vi "mapown org loop.vi"() -> ()   [LabVIEW 2011]
panel:
  in  "Close":bool
  in  "Update View":bool
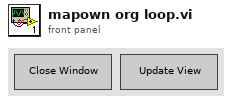
[diagram p1: front panel]
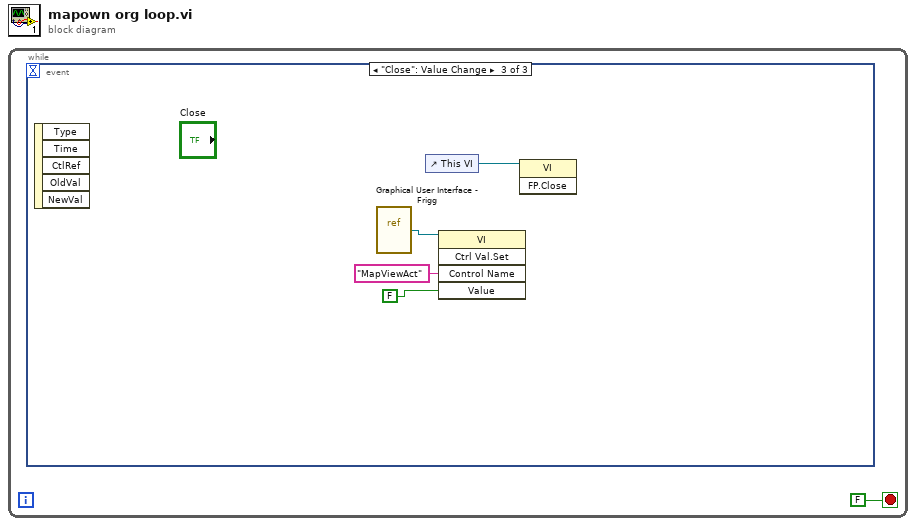
[diagram p0: block diagram]
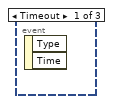
[diagram p2: hidden frame]
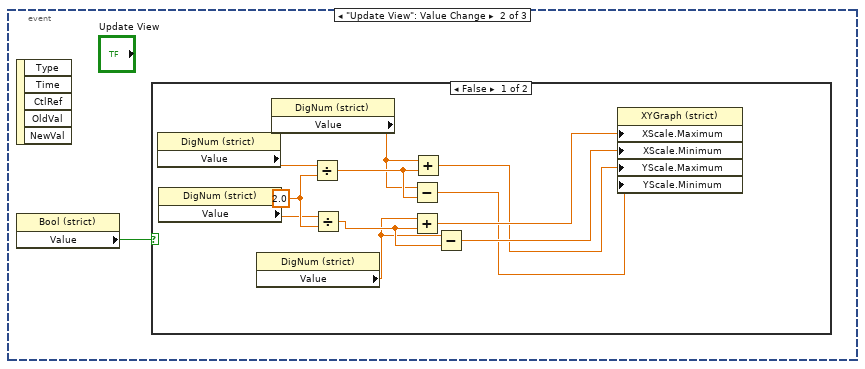
[diagram p3: hidden frame]
diagram:
  n1 = while {
    stop <- FALSE stop-if-true
    n2 = event shown="[2] \"Close\": Value Change" {
      selector: _ -> [_ _ _]
      dyn-events: _ -> [_ _ _]
      timeout: _ -> [_ _ _]
      event Timeout {
        n3 = event-data() -> ()  [unwired: 1 in, 2 out]
      }
      event "Update View": Value Change {
        n4 = event-data() -> ()  [unwired: 1 in, 5 out]
        n5 = property on="Property Node" class="Bool (strict)"() -> ("Value"=w2:bool)  [unwired: 2 in, 2 out]
        n6 = case shown="False" w2 {
          frame False {
            w13 = 2.0
            n7 = property on="Property Node" class="DigNum (strict)"() -> ("Value"=w5:dbl)  [unwired: 2 in, 2 out]
            n8 = property on="Property Node" class="DigNum (strict)"() -> ("Value"=w4:dbl)  [unwired: 2 in, 2 out]
            n9 = property on="Property Node" class="DigNum (strict)"() -> ("Value"=w3:dbl)  [unwired: 2 in, 2 out]
            n10 = property on="Property Node" class="DigNum (strict)"() -> ("Value"=w6:dbl)  [unwired: 2 in, 2 out]
            n11 = Divide(x=w5, y=w13) -> (x/y=w12:dbl)
            n12 = Divide(x=w4, y=w13) -> (x/y=w11:dbl)
            n13 = Subtract(x=w6, y=w12) -> (x-y=w7:dbl)
            n14 = Add(x=w3, y=w11) -> (x+y=w10:dbl)
            n15 = Add(x=w6, y=w12) -> (x+y=w8:dbl)
            n16 = Subtract(x=w3, y=w11) -> (x-y=w9:dbl)
            n17 = property on="Property Node" class="XYGraph (strict)"("XScale.Maximum"=w10, "XScale.Minimum"=w9, "YScale.Maximum"=w8, "YScale.Minimum"=w7) -> ()  [unwired: 2 in, 2 out]
          }
          frame True {
          }
        }
      }
      event "Close": Value Change {
        n18 = event-data() -> ()  [unwired: 1 in, 5 out]
        n19 = vi-ref "Graphical User Interface - Frigg.vi"() -> (w16:refnum<vi>)
        n20 = control-ref of="This VI"() -> (w17:refnum<vi>)
        n21 = invoke class="VI" method="Ctrl Val.Set"(reference=w16, "Control Name"="MapViewAct", "Value"=FALSE) -> ()  [unwired: 2 in, 5 out]
        n22 = invoke class="VI" method="FP.Close"(reference=w17) -> ()  [unwired: 2 in, 3 out]
      }
    }
  }
